vi "Main.vi"() -> ()   [LabVIEW 2021]
doc: "Use this template to build a simple state machine design pattern. Each state executes code and determines which state to transition to."
uses:
  controls/State.ctl
  <vilib>/Plasmionique/MB Master/MB_Master/MB_Master.lvclass
  <vilib>/Plasmionique/MB Master/MB_Master_TCP/MB_Master_TCP.lvclass
  C:/Program Files (x86)/National Instruments/LabVIEW 2021/vi.lib/Plasmionique/MB Master/MB_Master/MB_Master.lvclass
  <vilib>/Plasmionique/MB Master/MB Master.lvlib
  <vilib>/Analysis/NI_AALPro.lvlib
panel:
  out "Time Stamp":timestamp format="%<%H:%M:%S\n%d/%m/%y>T"
  in  "Tab Control":T1(tab)
  out "Nivel Alto":bool
  out "TQ - 01":dbl(slide) scale=0.0..100.0
  out "Vazão (L/s) 2":dbl
  out "BA - 01":bool
  out "FI - 01":dbl(knob) scale=0.0..100.0
  out "Nivel (Litros)":dbl format="%#_7g"
  out "Nivel Baixo":bool
  out "Alerta de vazão":bool
  out "Falha BA - 01":bool
  out "Nível Histórico":dbl[](graph)
  out "Vazão Histórica":dbl[](graph)
  in  "Configuração Hardware":T2={"IP Address"="", "Port"=502, "Slave ID"=1, "Timeout"=10000}
  out "MODBUS TCP/IP":bool
  in  "Conectar":bool
  in  "stop":bool
  # "Supervisório Abastecimento de Tanques"
  # "Diagrama operacional"
  # "Condominio"
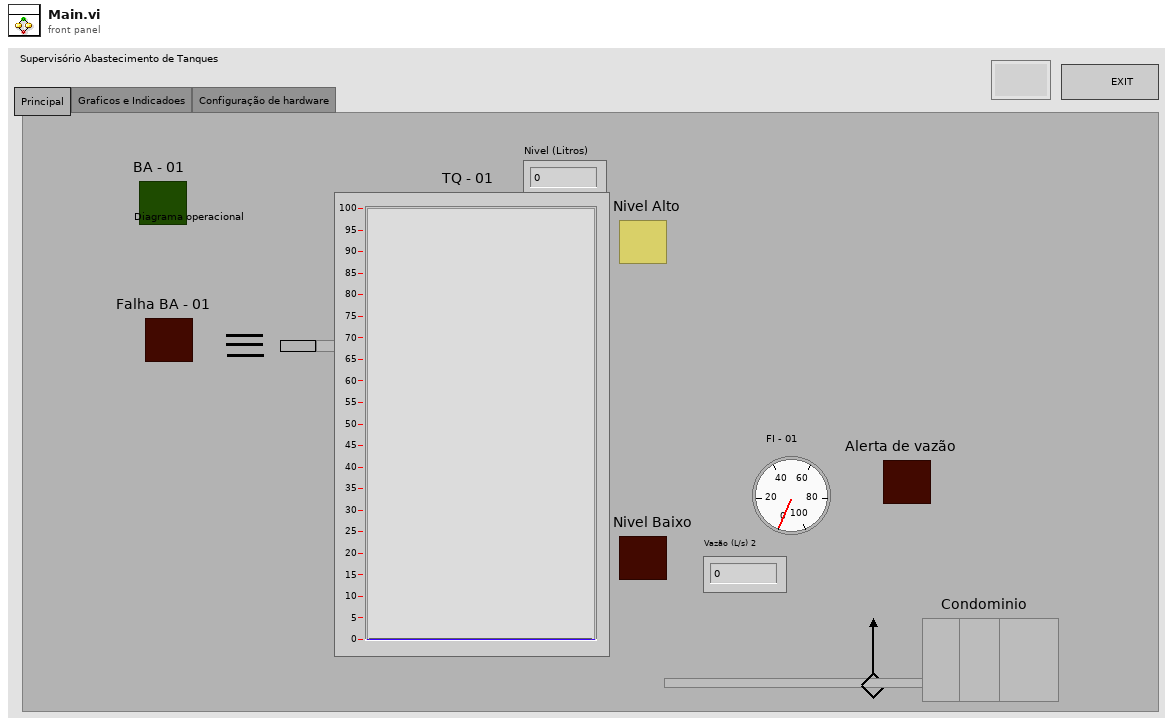
[diagram p1: front panel]
types:
  T1 = enum32{"Principal", "Graficos e Indicadoes", "Configuração de hardware"}
  T2 = cluster{"IP Address":string, "Port":u16, "Slave ID":u8, "Timeout":i32}
  T3 = enum8{"Enabled", "Disabled", "Disabled and Grayed Out"}
  T4 = typedef "State.ctl" = enum16{"Initialize", "Wait for Event", "Conectar", "Plota_dados", "Exit"}
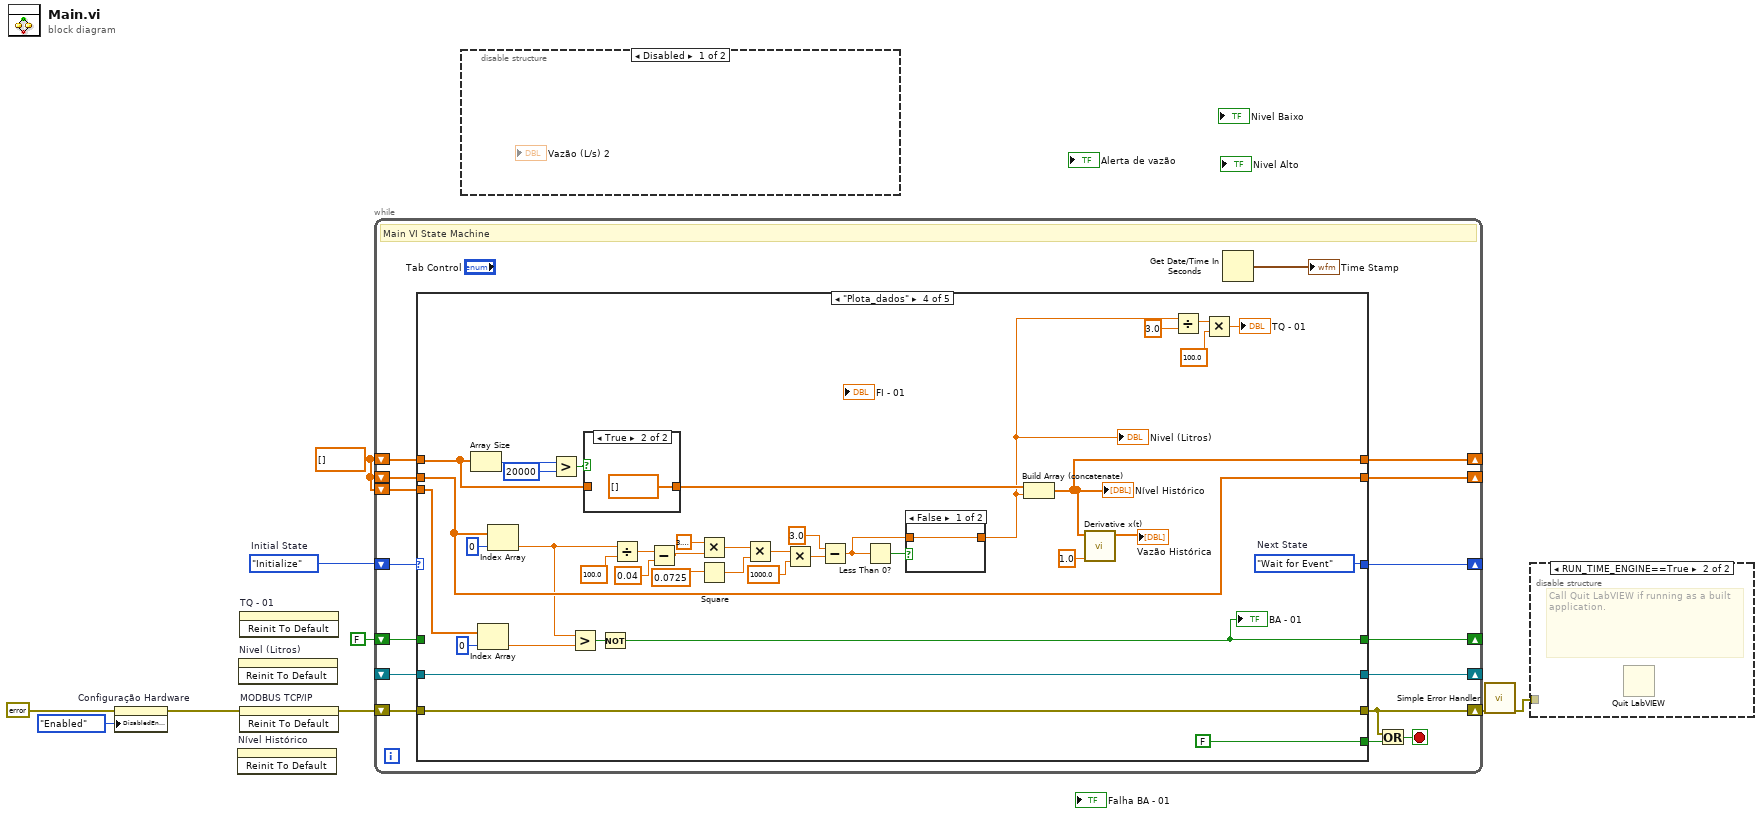
[diagram p0: block diagram]
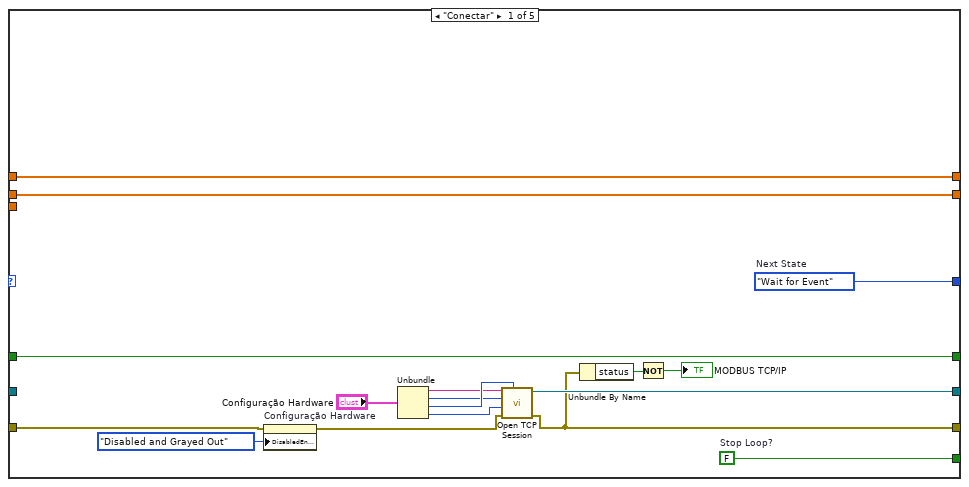
[diagram p4: hidden frame]
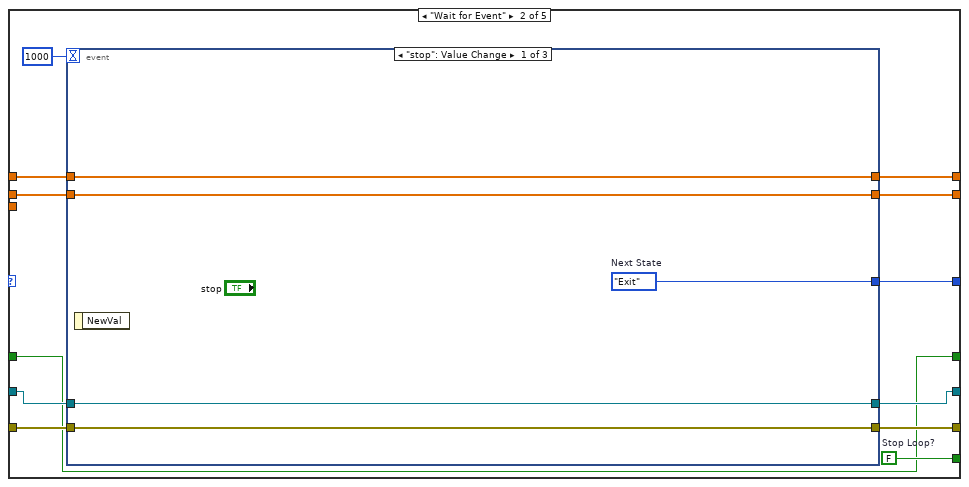
[diagram p5: hidden frame]
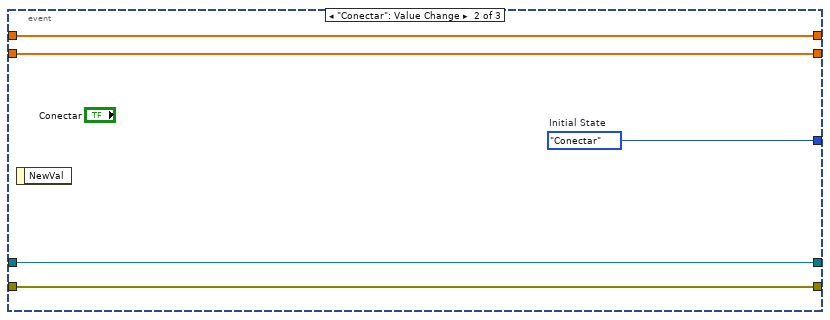
[diagram p6: hidden frame]
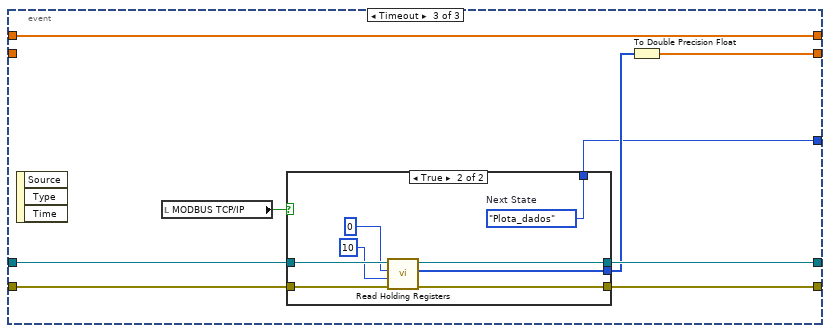
[diagram p7: hidden frame]
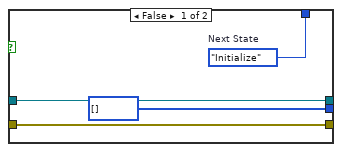
[diagram p8: hidden frame]
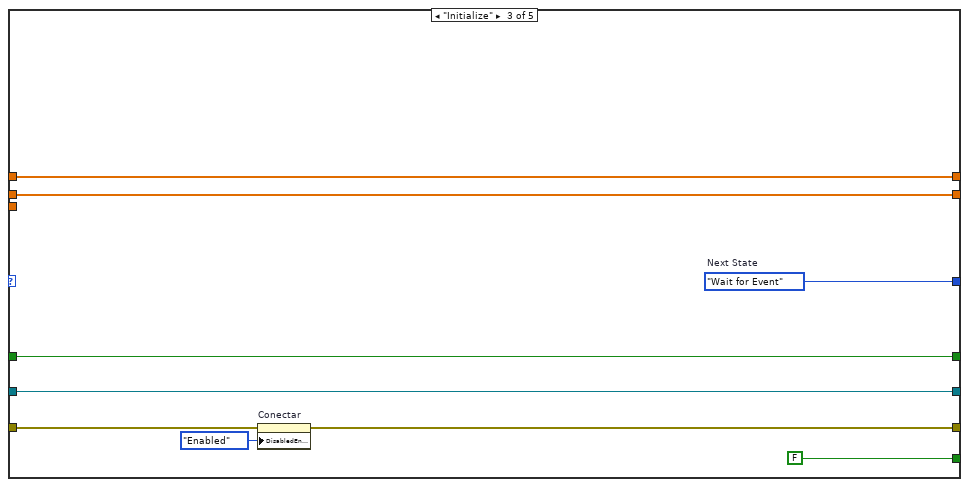
[diagram p9: hidden frame]
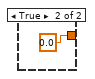
[diagram p10: hidden frame]
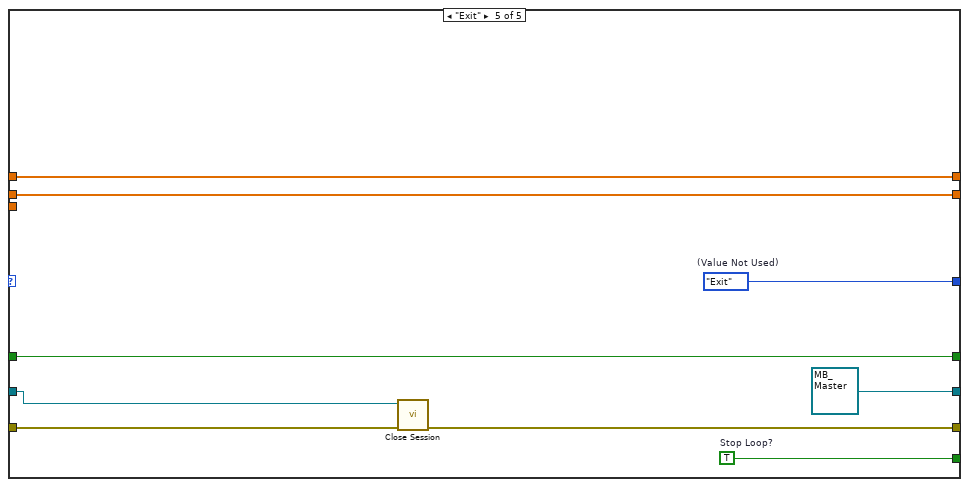
[diagram p12: hidden frame]
diagram:
  w2 = dbl[] []
  w9 = State."Initialize"  # Initial State
  n1 = property on="Configuração Hardware" class="Clust (strict)"(error in=errorcluster {"status"=FALSE, "code"=0, "source"=""} ("error constant"), "DisabledEnum"=T3."Enabled" ("Disabled")) -> (error out=w4:errorcluster)  [unwired: 1 in, 1 out]
  n2 = invoke on="Nível Histórico" class="WFGraph (strict)" method="Reinit To Default"() -> ()  [unwired: 3 in, 3 out]
  n3 = invoke on="Nivel (Litros)" class="DigNum (strict)" method="Reinit To Default"() -> ()  [unwired: 3 in, 3 out]
  n4 = invoke on="TQ - 01" class="Slide (strict)" method="Reinit To Default"() -> ()  [unwired: 3 in, 3 out]
  n5 = invoke on="MODBUS TCP/IP" class="Bool (strict)" method="Reinit To Default"(error in=w4) -> (error out=w3:errorcluster)  [unwired: 2 in, 2 out]
  n6 = while {
    shift-right: [w24] -> _
    shift-left: w9 -> [w25]
    shift-right: [w20] -> w8
    shift-left: w3 -> [w23]
    shift-right: [w19] -> _
    shift-left: _ -> [w18]
    shift-right: [w16] -> _
    shift-left: w2 -> [w17]
    shift-right: [w14] -> _
    shift-left: w2 -> [w13]
    shift-left: w2 -> [w12]
    shift-right: [w10] -> _
    shift-left: FALSE -> [w11]
    stop <- w21 stop-if-true
    # "Main VI State Machine"
    n7 = case shown="\"Plota_dados\"" w25 {
      tunnel: [w42 w54 w94 w133 w146] -> w24
      tunnel: [w41 w53 FALSE ("Stop Loop?") FALSE ("Stop Loop?") w145] -> w22
      tunnel: w23 -> [w33 w52 w89 w131 w144]
      tunnel: [w31 w51 w88 w131 w143] -> w20
      tunnel: [w35 w49 w92 w130 refnum<class "MB_Master.lvclass"> refnum ("MB session out")] -> w19
      tunnel: w18 -> [_ w48 w92 w130 w142]
      tunnel: w17 -> [w28 w47 w91 w109 w140]
      tunnel: [w28 w46 w91 w97 w140] -> w16
      tunnel: [w27 w45 w90 w107 w139] -> w14
      tunnel: w13 -> [w27 w44 w90 w107 w139]
      tunnel: w12 -> [_ _ _ w102 _]
      tunnel: [w26 w43 w86 w100 w138] -> w10
      tunnel: w11 -> [w26 w43 w86 _ w138]
      frame "Conectar" {
        w41 = FALSE  # Stop Loop?
        w42 = State."Wait for Event"  # Next State
        # "Initialize - Initialize the application."
        n8 = property on="Configuração Hardware" class="Clust (strict)"(error in=w33, "DisabledEnum"=T3."Disabled and Grayed Out" ("Disabled")) -> (error out=w32:errorcluster)  [unwired: 1 in, 1 out]
        n9 = Unbundle("Configuração Hardware") -> ("IP Address"=w39:string, "Port"=w38:u16, "Slave ID"=w40:u8, "Timeout"=w37:i32)
        n10 = call <vilib>:"Open TCP Session.vi"("Slave ID (255)"=w40, "error in (no error)"=w32, "Timeout (10000)"=w37, "Port (502)"=w38, "IP Address"=w39) -> ("error out"=w31:errorcluster, "MB_TCP session"=w35:refnum<class "MB_Master_TCP.lvclass">)  [unwired: 5 in]
        n11 = Unbundle By Name(w31) -> ("status"=w30:bool)
        n12 = Not(x=w30) -> (.not. x?=→"MODBUS TCP/IP":bool)
      }
      frame "Wait for Event" {
        w53 = FALSE  # Stop Loop?
        # "Wait for Event - Use an Event Structure to monitor the user interface for events that run different states of the state machine."
        n13 = event shown="[0] \"stop\": Value Change" {
          selector: _ -> [_ _ _]
          dyn-events: _ -> [_ _ _]
          timeout: 1000 -> [_ _ _]
          tunnel: [w58 w63 w65] -> w54
          tunnel: w52 -> [w59 w64 w73]
          tunnel: [w59 w64 w72] -> w51
          tunnel: [w57 w62 w71] -> w49
          tunnel: w48 -> [w57 w62 w70]
          tunnel: w47 -> [w56 w61 w69]
          tunnel: [w56 w61 w69] -> w46
          tunnel: [w55 w60 w67] -> w45
          tunnel: w44 -> [w55 w60 _]
          event "stop": Value Change {
            w58 = State."Exit"  # Next State
            n14 = event-data() -> ()  [unwired: 1 in, 1 out]
          }
          event "Conectar": Value Change {
            w63 = State."Conectar"  # Initial State
            n15 = event-data() -> ()  [unwired: 1 in, 1 out]
          }
          event Timeout {
            n16 = event-data() -> ()  [unwired: 1 in, 3 out]
            n17 = local read "MODBUS TCP/IP"() -> (w66:bool)
            n18 = case shown="True" w66 {
              tunnel: w73 -> [w76 w85]
              tunnel: [w76 w84] -> w72
              tunnel: [w77 w83] -> w71
              tunnel: w70 -> [w77 w82]
              tunnel: [u16[] [] ("Registers") w79] -> w68
              tunnel: [w74 w78] -> w65
              frame False {
                w74 = State."Initialize"  # Next State
              }
              frame True {
                w78 = State."Plota_dados"  # Next State
                n19 = call <vilib>:"Read Holding Registers.vi"("error in (no error)"=w85, "quantity"=u16 10, "starting address"=u16 0, "MB session in"=w82) -> ("error out"=w84:errorcluster, "Registers"=w79:u16[], "MB session out"=w83:refnum<class "MB_Master.lvclass">)  [unwired: 5 in]
              }
            }
            n20 = To Double Precision Float(number=w68) -> (double precision float=w67:dbl[])
          }
        }
      }
      frame "Initialize" {
        w94 = State."Wait for Event"  # Next State
        n21 = property on="Conectar" class="Bool"(error in=w89, "DisabledEnum"=T3."Enabled" ("Disabled")) -> (error out=w88:errorcluster)  [unwired: 1 in, 1 out]
      }
      frame "Plota_dados" {
        w133 = State."Wait for Event"  # Next State
        # "User State 2 - Replace this state with functionality for your own application."
        n22 = Array Size(array=w109) -> (size(s)=w121:i32)
        n23 = Index Array(array=w102, index=0) -> (element=w98:dbl)
        n24 = Index Array(array=w107, index=0) -> (element=w99:dbl)
        n25 = Greater?(x=w121, y=20000) -> (0:w119:bool)
        n26 = Greater?(x=w99, y=w98) -> (0:w101:bool)
        n27 = case shown="True" w119 {
          tunnel: w109 -> [w136 _]
          tunnel: [w136 dbl[] []] -> w110
          frame False {
          }
          frame True {
          }
        }
        n28 = Not(x=w101) -> (.not. x?=w100:bool)
        "BA - 01" <- w100
        n29 = Divide(x=w99, y=100.0) -> (x/y=w117:dbl)
        n30 = Subtract(x=w117, y=0.04) -> (x-y=w116:dbl)
        n31 = Multiply(x=3.141592653589793, y=w116) -> (x*y=w128:dbl)
        n32 = Square(x=0.0725) -> (x^2=w127:dbl)
        n33 = Multiply(x=w128, y=w127) -> (x*y=w125:dbl)
        n34 = Multiply(x=w125, y=1000.0) -> (x*y=w115:dbl)
        n35 = Subtract(x=3.0 ("y"), y=w115) -> (x-y=w105:dbl)
        n36 = Less Than 0?(x=w105) -> (x < 0?=w106:bool)
        n37 = case shown="False" w106 {
          tunnel: w105 -> [w134 _]
          tunnel: [w134 0.0] -> w104
          frame False {
          }
          frame True {
          }
        }
        "Nivel (Litros)" <- w104
        n38 = Build Array (concatenate)(w110, w104) -> (w97:dbl[])
        "Nível Histórico" <- w97
        n39 = call <vilib>:"Derivative x(t).vi"("dt"=1.0, "X"=w97) -> ("dX/dt"=→"Vazão Histórica":dbl[])  [unwired: 8 in, 1 out]
        n40 = Divide(x=w104, y=3.0) -> (x/y=w113:dbl)
        n41 = Multiply(x=w113, y=100.0) -> (x*y=→"TQ - 01":dbl)
      }
      frame "Exit" {
        w145 = TRUE  # Stop Loop?
        w146 = State."Exit"  # (Value Not Used)
        # "Exit - Exit the application."
        n42 = call-dynamic "Close Session.vi"("error in (no error)"=w144, "MB session in"=w142) -> ("error out"=w143:errorcluster)  [unwired: 9 in]
      }
    }
    n43 = Get Date/Time In Seconds() -> (seconds since 1Jan1904=→"Time Stamp":timestamp)
    n44 = Or(x=w20, y=w22) -> (x .or. y?=w21:bool)
  }
  n45 = disable-structure shown="Disabled" {
    frame Disabled {
    }
    frame Enabled {
    }
  }
  n46 = call <vilib>:"Simple Error Handler.vi"("error in (no error)"=w8) -> ("error out"=w7:errorcluster)  [unwired: 4 in, 4 out]
  n47 = disable-structure shown="RUN_TIME_ENGINE==True" {
    disable-tunnel: w7 -> [_ _]
    frame condition #0 (active) {
    }
    frame condition #1 {
      # "Call Quit LabVIEW if running as a built application."
      n48 = Quit LabVIEW() -> ()  [unwired: 1 in]
    }
  }
